vi "Read Pin Map.vi"(8 "error in (no error)":errorcluster, 11 "NI-DAQ in":refnum<class "NI-DAQ.lvclass">) -> (0 "error out":errorcluster, 2 "Pin Map":T1={"Region Valves"=[49, 52, 0, 0], "Extra Valves"=[[[0.0, 48.0, 0.0, 0.0, 0.0]]], "Tool Primary Valve"=51, "Tool Secondary Valve"=50, "Region Sensors"=[37, 41, 37], "Extra Sensors"=[[[36.0, 37.0, 0.0, 0.0]]], "Tool Primary Sensor"=39.0, "Tool Secondary Sensor"=38.0, "Compression Sensor"=31.0, "5V"=50}, 3 "NI-DAQ out":refnum<class "NI-DAQ.lvclass">)   [LabVIEW 2016, in "NI-DAQ.lvclass"]
uses:
  NI-DAQ.lvclass
  Pin Map.ctl
  I-O.lvclass
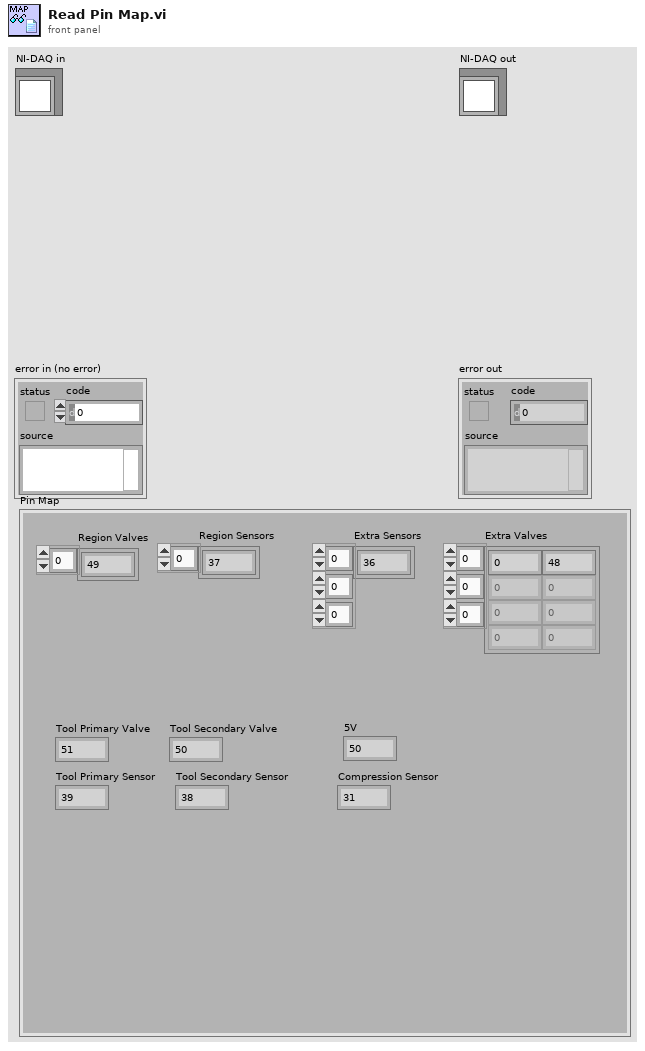
[diagram p1: front panel]
types:
  T1 = typedef "I-O.lvclass/Pin Map.ctl" = cluster{"Region Valves":i32[], "Extra Valves":dbl[][][], "Tool Primary Valve":i32, "Tool Secondary Valve":i32, "Region Sensors":i32[], "Extra Sensors":dbl[][][], "Tool Primary Sensor":dbl, "Tool Secondary Sensor":dbl, "Compression Sensor":dbl, "5V":i32}
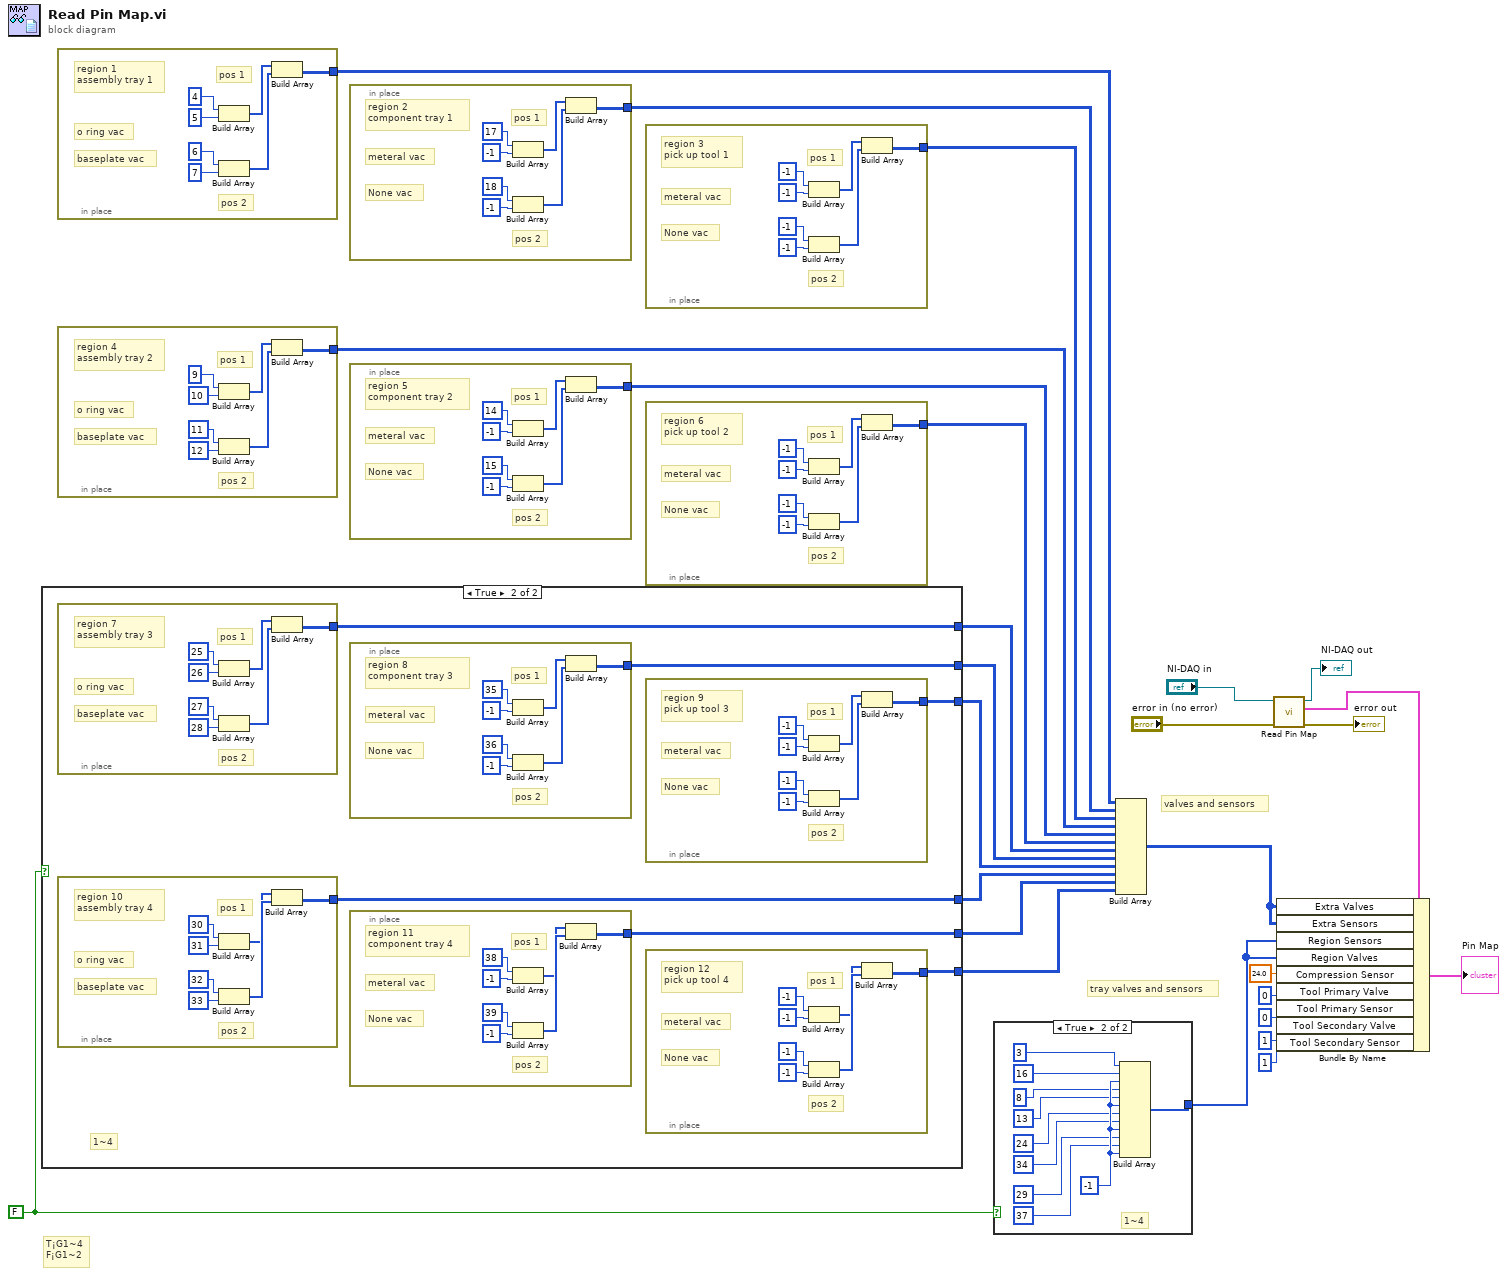
[diagram p0: block diagram]
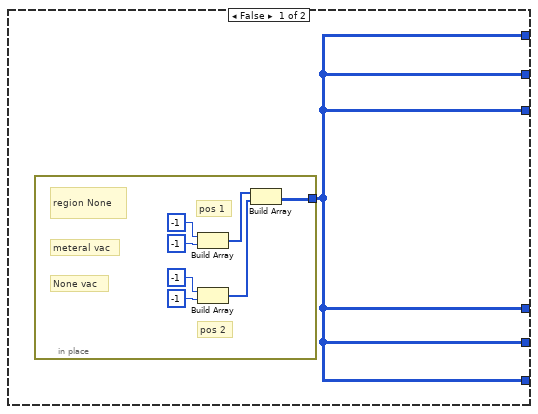
[diagram p2: hidden frame]
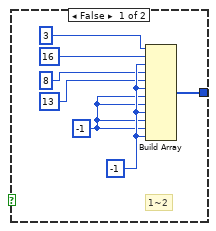
[diagram p3: hidden frame]
diagram:
  w1 = FALSE
  # "T¡G1~4\nF¡G1~2"
  # "tray valves and sensors"
  # "valves and sensors"
  n1 = case shown="True" w1 {
    tunnel: [w27 w40] -> w8
    tunnel: [w27 w39] -> w7
    tunnel: [w27 w38] -> w6
    tunnel: [w27 w37] -> w5
    tunnel: [w27 w36] -> w4
    tunnel: [w27 w35] -> w3
    frame False {
      n2 = in-place {
        in-place-border: [w28] -> w27
        # "region None"
        # "pos 2"
        # "None vac"
        # "meteral vac"
        # "pos 1"
        n3 = Build Array(-1, -1) -> (w29:i32[])
        n4 = Build Array(-1, -1) -> (w30:i32[])
        n5 = Build Array(w29, w30) -> (w28:i32[][])
      }
    }
    frame True {
      # "1~4"
      n6 = in-place {
        in-place-border: [w76] -> w40
        # "region 7\nassembly tray 3"
        # "pos 2"
        # "baseplate vac"
        # "o ring vac"
        # "pos 1"
        n7 = Build Array(25, 26) -> (w77:i32[])
        n8 = Build Array(27, 28) -> (w78:i32[])
        n9 = Build Array(w77, w78) -> (w76:i32[][])
      }
      n10 = in-place {
        in-place-border: [w55] -> w37
        # "region 10\nassembly tray 4"
        # "pos 2"
        # "baseplate vac"
        # "o ring vac"
        # "pos 1"
        n11 = Build Array(30, 31) -> (w56:i32[])
        n12 = Build Array(32, 33) -> (w57:i32[])
        n13 = Build Array(w56, w57) -> (w55:i32[][])
      }
      n14 = in-place {
        in-place-border: [w69] -> w39
        # "region 8\ncomponent tray 3"
        # "pos 2"
        # "None vac"
        # "meteral vac"
        # "pos 1"
        n15 = Build Array(35, -1) -> (w70:i32[])
        n16 = Build Array(36, -1) -> (w71:i32[])
        n17 = Build Array(w70, w71) -> (w69:i32[][])
      }
      n18 = in-place {
        in-place-border: [w48] -> w36
        # "region 11\ncomponent tray 4"
        # "pos 2"
        # "None vac"
        # "meteral vac"
        # "pos 1"
        n19 = Build Array(38, -1) -> (w49:i32[])
        n20 = Build Array(39, -1) -> (w50:i32[])
        n21 = Build Array(w49, w50) -> (w48:i32[][])
      }
      n22 = in-place {
        in-place-border: [w62] -> w38
        # "region 9\npick up tool 3"
        # "pos 2"
        # "None vac"
        # "meteral vac"
        # "pos 1"
        n23 = Build Array(-1, -1) -> (w63:i32[])
        n24 = Build Array(-1, -1) -> (w64:i32[])
        n25 = Build Array(w63, w64) -> (w62:i32[][])
      }
      n26 = in-place {
        in-place-border: [w41] -> w35
        # "region 12\npick up tool 4"
        # "pos 2"
        # "None vac"
        # "meteral vac"
        # "pos 1"
        n27 = Build Array(-1, -1) -> (w42:i32[])
        n28 = Build Array(-1, -1) -> (w43:i32[])
        n29 = Build Array(w42, w43) -> (w41:i32[][])
      }
    }
  }
  n30 = in-place {
    in-place-border: [w83] -> w15
    # "region 1\nassembly tray 1"
    # "pos 2"
    # "baseplate vac"
    # "o ring vac"
    # "pos 1"
    n31 = Build Array(4, 5) -> (w84:i32[])
    n32 = Build Array(6, 7) -> (w85:i32[])
    n33 = Build Array(w84, w85) -> (w83:i32[][])
  }
  n34 = in-place {
    in-place-border: [w90] -> w11
    # "region 4\nassembly tray 2"
    # "pos 2"
    # "baseplate vac"
    # "o ring vac"
    # "pos 1"
    n35 = Build Array(9, 10) -> (w91:i32[])
    n36 = Build Array(11, 12) -> (w92:i32[])
    n37 = Build Array(w91, w92) -> (w90:i32[][])
  }
  n38 = in-place {
    in-place-border: [w97] -> w13
    # "region 2\ncomponent tray 1"
    # "pos 2"
    # "None vac"
    # "meteral vac"
    # "pos 1"
    n39 = Build Array(17, -1) -> (w98:i32[])
    n40 = Build Array(18, -1) -> (w99:i32[])
    n41 = Build Array(w98, w99) -> (w97:i32[][])
  }
  n42 = in-place {
    in-place-border: [w104] -> w10
    # "region 5\ncomponent tray 2"
    # "pos 2"
    # "None vac"
    # "meteral vac"
    # "pos 1"
    n43 = Build Array(14, -1) -> (w105:i32[])
    n44 = Build Array(15, -1) -> (w106:i32[])
    n45 = Build Array(w105, w106) -> (w104:i32[][])
  }
  n46 = in-place {
    in-place-border: [w111] -> w12
    # "region 3\npick up tool 1"
    # "pos 2"
    # "None vac"
    # "meteral vac"
    # "pos 1"
    n47 = Build Array(-1, -1) -> (w112:i32[])
    n48 = Build Array(-1, -1) -> (w113:i32[])
    n49 = Build Array(w112, w113) -> (w111:i32[][])
  }
  n50 = in-place {
    in-place-border: [w118] -> w9
    # "region 6\npick up tool 2"
    # "pos 2"
    # "None vac"
    # "meteral vac"
    # "pos 1"
    n51 = Build Array(-1, -1) -> (w119:i32[])
    n52 = Build Array(-1, -1) -> (w120:i32[])
    n53 = Build Array(w119, w120) -> (w118:i32[][])
  }
  n54 = case shown="True" w1 {
    tunnel: [w125 w132] -> w2
    frame False {
      w126 = -1
      w129 = -1
      # "1~2"
      n55 = Build Array(3, 16, w129, 8, 13, w129, w126, w126, w129, w126, w126, w129) -> (w125:i32[])
    }
    frame True {
      w139 = -1
      # "1~4"
      n56 = Build Array(3, 16, w139, 8, 13, w139, 24, 34, w139, 29, 37, w139) -> (w132:i32[])
    }
  }
  n57 = Build Array(w15, w13, w12, w11, w10, w9, w8, w7, w6, w5, w4, w3) -> (w14:i32[][][])
  n58 = call-parent "Read Pin Map.vi"("error in (no error)"="error in (no error)", "I-O in"="NI-DAQ in") -> ("error out"=→"error out":errorcluster, "Pin Map 2"=w22:T1, "I-O out"=→"NI-DAQ out":refnum<class "NI-DAQ.lvclass">)  [unwired: 7 in]
  n59 = Bundle By Name(cluster=w22, "Extra Valves"=w14, "Extra Sensors"=w14, "Region Sensors"=w2, "Region Valves"=w2, "Compression Sensor"=24.0, "Tool Primary Valve"=0, "Tool Primary Sensor"=0 ("Tool Primary Valve"), "Tool Secondary Valve"=1 ("Tool Primary Valve"), "Tool Secondary Sensor"=1 ("Tool Secondary Valve")) -> (→"Pin Map":T1)
